vi "Auto Drive.vi"(6 "Reinitialize":bool, 8 "Strafe target":dbl, 9 "Heading target":dbl, 10 "Y target":dbl) -> (0 "X out":dbl, 1 "Strafe out":dbl, 2 "Y out":dbl, 3 "isFinished":bool)   [LabVIEW 2014]
uses:
  Common Code/Change Detect Double.vi
  Robot Global Data.vi
panel:
  in  "Max Stop Speed":dbl
  in  "Distance Stop Threshold":dbl
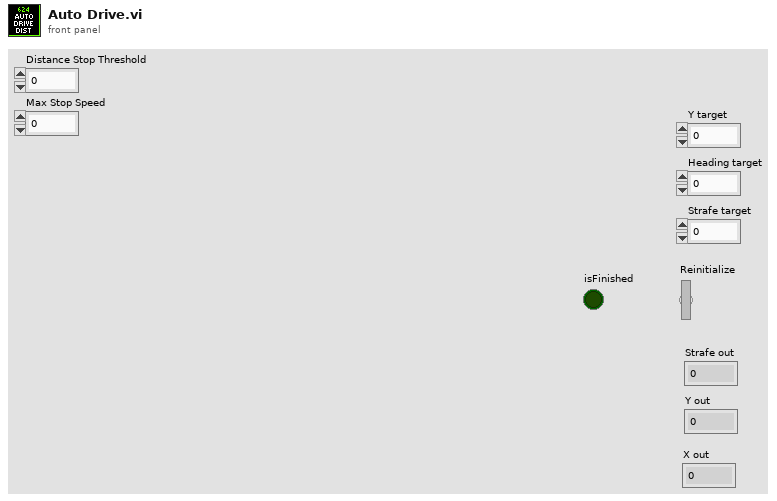
[diagram p1: front panel]
types:
  T1 = typedef "Dashboard Control Data.ctl" = cluster{"Cam Exposure":dbl, "Go to angle":dbl, "Steer PID Gains":cluster{"proportional gain (Kc)":dbl, "integral time (Ti, min)":dbl, "derivative time (Td, min)":dbl}, "Steer PID output Range":cluster{"output high":dbl, "output low":dbl}, "Pressure m \nValue":dbl, "Pressure b \nValue":dbl, "Strafe Timer\nWait":dbl, "Roller Command Cluster ":T2, "Elevator":T3, "Strafe Correct max steer":dbl, "IMU Enable":bool, "Encoder Control":T5, "IMU Controls":cluster{"Pitch Zero":dbl, "Roll Zero":dbl}, "Auton Settings":cluster{"Drive Dist Window Size":dbl}}
  T2 = typedef "Roller Control.ctl" = cluster{"Intake Speed":dbl, "Turn In Speed":dbl, "Unload Speed":dbl, "Turn Out Speed":dbl, "Ping Align Tolerance":dbl, "Tote Range Threshold":dbl, "Right Pot 0":dbl, "Pot Threshold":dbl, "Left Pot 0":dbl, "Manual 0s?":bool, "Right Pot Scale":dbl, "Left Pot Scale":dbl, "0 wait time":i32, "Zero Pots":bool, "Min Elevator Height":dbl, "Eject Time":dbl, "Eject US Threshold":dbl, "Anti-Twitch Time":u32, "Ping Caring Threshold":dbl, "Pot Diff Threshold":dbl, "Pinch Sustain":u32, "Absorb Give Up Threshold":dbl, "Untip In Threshold":dbl, "Untip Grab Range":dbl}
  T3 = typedef "Elevator DB Control.ctl" = cluster{"PID Output Range":cluster{"output high":dbl, "output low":dbl}, "PID gains":cluster{"proportional gain (Kc)":dbl, "integral time (Ti, min)":dbl, "derivative time (Td, min)":dbl}, "Height Tolerance":sgl, " Encoder Constant":dbl, "Safe Mode Max Speed":sgl, "Eject Time":sgl, "Zeroing Speed":sgl, "Presets":T4, "Ping Detect Threshold":sgl, "Trashcan Detect Threshold":sgl, "Zero Filter Time":dbl, "Stabilizer Open Time":dbl}
  T4 = typedef "Elevator Presets.ctl" = cluster{"Hold Tote":sgl, "Hold Trashcan":sgl, "Pickup 2 w/ Tote":sgl, "Pickup 2 w/ Trashcan":sgl, "Pickup 3 w/ Tote":sgl, "Pickup 3 w/ Trashcan":sgl, "Bottom":sgl, "Pickup 1 w/ Tote":sgl, "Pickup Trashcan":sgl, "Pickup 1 w/ Trashcan":sgl, "Eject":sgl, "Hold Low":sgl, "Step add height":sgl, "Store Trashcan 3":sgl, "Store Trashcan 4":sgl, "Store Trashcan 5":sgl, "6 Tote Max Height":sgl, "5 Tote Max Height":sgl, "Idle Empty":dbl, "Untip Lift":dbl, "Drop Stack":dbl}
  T5 = typedef "Encoder Control.ctl" = cluster{"Left Tick Constant":dbl, "Right Tick Constant":dbl, "Center Tick Constant":dbl, "Reset?":bool, "Y Dist":cluster{"PID gains":cluster{"proportional gain (Kc)":dbl, "integral time (Ti, min)":dbl, "derivative time (Td, min)":dbl}, "output range":cluster{"output high":dbl, "output low":dbl}}, "X Dist":cluster{"PID gains":cluster{"proportional gain (Kc)":dbl, "integral time (Ti, min)":dbl, "derivative time (Td, min)":dbl}, "output range":cluster{"output high":dbl, "output low":dbl}}, "Y Stop Thresh":dbl, "Y Stop Speed":dbl, "X Stop Thresh":dbl, "X Stop Speed":dbl}
  T6 = typedef "Encoder Values SuperCluster.ctl" = cluster{"Left Encoder":T7, "Center Encoder":T7, "Right Encoder":T7}
  T7 = typedef "Encoder Values.ctl" = cluster{"Distance":dbl, "Speed":dbl, "Ticks":dbl}
  T8 = cluster{"PID gains":cluster{"proportional gain (Kc)":dbl, "integral time (Ti, min)":dbl, "derivative time (Td, min)":dbl}, "output range":cluster{"output high":dbl, "output low":dbl}}
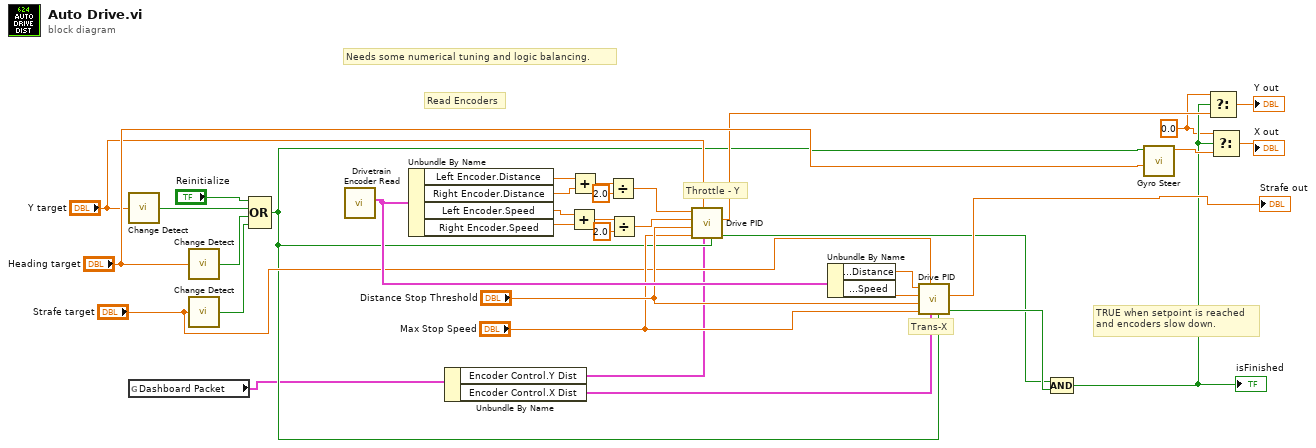
[diagram p0: block diagram]
diagram:
  w7 = 0.0 ("t")
  # "Throttle - Y"
  # "Trans-X"
  # "Needs some numerical tuning and logic balancing."
  # "Read Encoders"
  # "TRUE when setpoint is reached\nand encoders slow down."
  n1 = call-poly "Change Detect.vi"("In"="Y target") -> ("Changed?"=w35:bool)
  n2 = global read "Robot Global Data.vi" "Dashboard Packet"() -> (w3:T1)
  n3 = call-poly "Change Detect.vi"("In"="Heading target") -> ("Changed?"=w34:bool)
  n4 = call-poly "Change Detect.vi"("In"="Strafe target") -> ("Changed?"=w33:bool)
  n5 = Compound Arithmetic op=OR("Reinitialize", w35, w34, w33) -> (w4:bool)
  n6 = call "Drivetrain Encoder Read.vi"() -> ("Quick use cluster"=w26:T6)  [unwired: 11 in]
  n7 = Unbundle By Name(w26) -> ("Left Encoder.Distance"=w19:dbl, "Right Encoder.Distance"=w20:dbl, "Left Encoder.Speed"=w22:dbl, "Right Encoder.Speed"=w21:dbl)
  n8 = Unbundle By Name(w3) -> ("Encoder Control.Y Dist"=w2:T8, "Encoder Control.X Dist"=w1:T8)
  n9 = Add(x=w22, y=w21) -> (x+y=w15:dbl)
  n10 = Add(x=w19, y=w20) -> (x+y=w18:dbl)
  n11 = Divide(x=w18, y=2.0) -> (x/y=w14:dbl)
  n12 = Divide(x=w15, y=2.0) -> (x/y=w13:dbl)
  n13 = call "Drive PID.vi"("reinitialize? (F)"=w4, "PID Params"=w2, "Setpoint"="Y target", "Max Stop Speed"="Max Stop Speed", "Distance Stop Threshold"="Distance Stop Threshold", "Current Speed"=w13, "Current Distance"=w14) -> ("Finished"=w29:bool, "output"=w10:dbl)  [unwired: 3 in]
  n14 = Unbundle By Name(w26) -> ("Center Encoder.Distance"=w5:dbl, "Center Encoder.Speed"=w6:dbl)
  n15 = call "Drive PID.vi"("reinitialize? (F)"=w4, "PID Params"=w1, "Setpoint"="Strafe target", "Max Stop Speed"="Max Stop Speed", "Distance Stop Threshold"="Distance Stop Threshold", "Current Speed"=w6, "Current Distance"=w5) -> ("Finished"=w30:bool, "output"=→"Strafe out":dbl)  [unwired: 3 in]
  n16 = Compound Arithmetic op=AND(w29, w30) -> (w8:bool)
  "isFinished" <- w8
  n17 = call "Gyro Steer.vi"("Target Angle"="Heading target", "Changed?"=w4) -> ("X out"=w9:dbl)  [unwired: 9 in]
  n18 = Select(t=w7, s=w8, f=w10) -> (s? t:f=→"Y out":dbl)
  n19 = Select(t=w7, s=w8, f=w9) -> (s? t:f=→"X out":dbl)
